vi "Start Logging.vi"(8 "error in (no error)":errorcluster, 10 "Path":path, 11 "Data Logger Interface in":refnum<class "Data Logger Actor Interface.lvclass">) -> (0 "error out":errorcluster, 3 "Data Logger Interface out":refnum<class "Data Logger Actor Interface.lvclass">)   [LabVIEW 2024, in "Data Logger Actor Interface.lvlib" / "Data Logger Actor Interface.lvclass"]
uses:
  Data Logger Actor Interface.lvclass
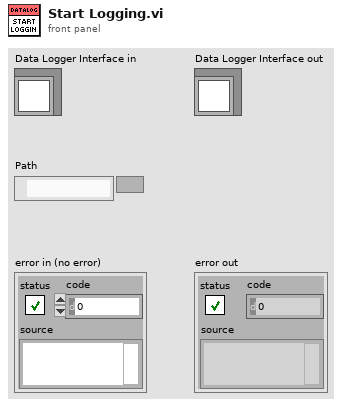
[diagram p1: front panel]
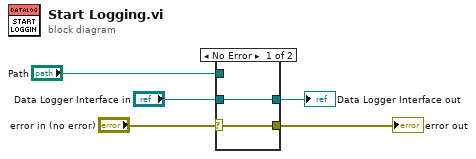
[diagram p0: block diagram]
diagram:
  n1 = case shown="No Error" "error in (no error)" {
    selector: "error in (no error)" -> [w6 w9]
    tunnel: [w6 w9] -> w4
    tunnel: [w7 w8] -> w2
    tunnel: "Data Logger Interface in" -> [w7 w8]
    tunnel: "Path" -> [_ _]
    frame No Error {
    }
    frame Error {
    }
  }
  "error out" <- w4
  "Data Logger Interface out" <- w2
